vi "Create End-of-shift Report.vi"(6 "Tesla per Amp":dbl format="%#_13g", 7 "MV/m per Probe Volt":dbl format="%#_13g", 8 "error in (no error)":errorcluster, 10 "Shift Start Time":T1, 11 "Parsed Pulse Data":T2(array[cluster])) -> (0 "error out":errorcluster, 3 "Log Entry Text":string)   [LabVIEW 2013, in "Controls Log Monitor.lvlib"]
uses:
  Controls Log Monitor.lvlib
  <vilib>/Utility/miscctls.llb/LVDateTimeRec.ctl
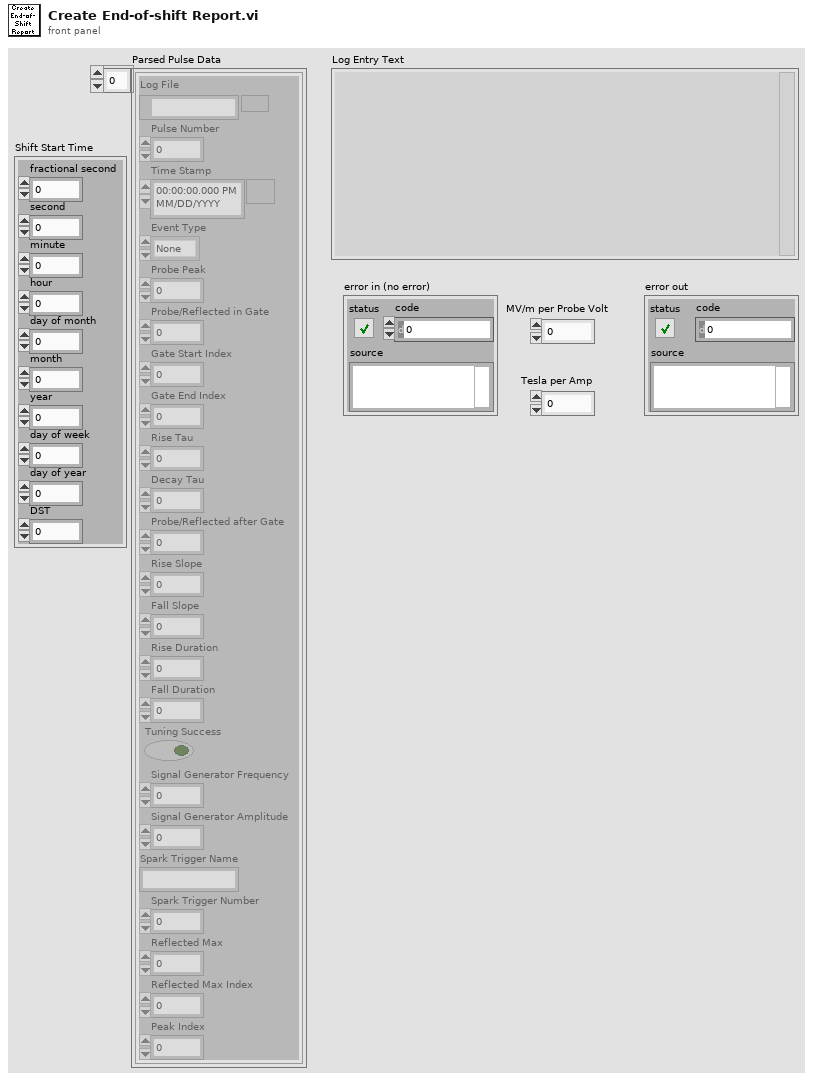
[diagram p1: front panel]
types:
  T1 = typedef "LVDateTimeRec.ctl" = cluster{"fractional second":dbl, "second":i32, "minute":i32, "hour":i32, "day of month":i32, "month":i32, "year":i32, "day of week":i32, "day of year":i32, "DST":i32}
  T2 = cluster{"Log File":path, "Pulse Number":u32, "Time Stamp":timestamp, "Event Type":enum16{"None", "Tune", "Periodic Capture", "Spark Trigger"}, "Probe Peak":dbl, "Probe/Reflected in Gate":dbl, "Gate Start Index":i32, "Gate End Index":i32, "Rise Tau":dbl, "Decay Tau":dbl, "Probe/Reflected after Gate":dbl, "Rise Slope":dbl, "Fall Slope":dbl, "Rise Duration":dbl, "Fall Duration":dbl, "Tuning Success":bool, "Signal Generator Frequency":dbl, "Signal Generator Amplitude":dbl, "Spark Trigger Name":string, "Spark Trigger Number":i32, "Reflected Max":dbl, "Reflected Max Index":i32, "Peak Index":i32}[]
  T3 = enum16{"None", "Tune", "Periodic Capture", "Spark Trigger"}
  T4 = cluster{"Name":string, "Value":dbl, "Units":string}
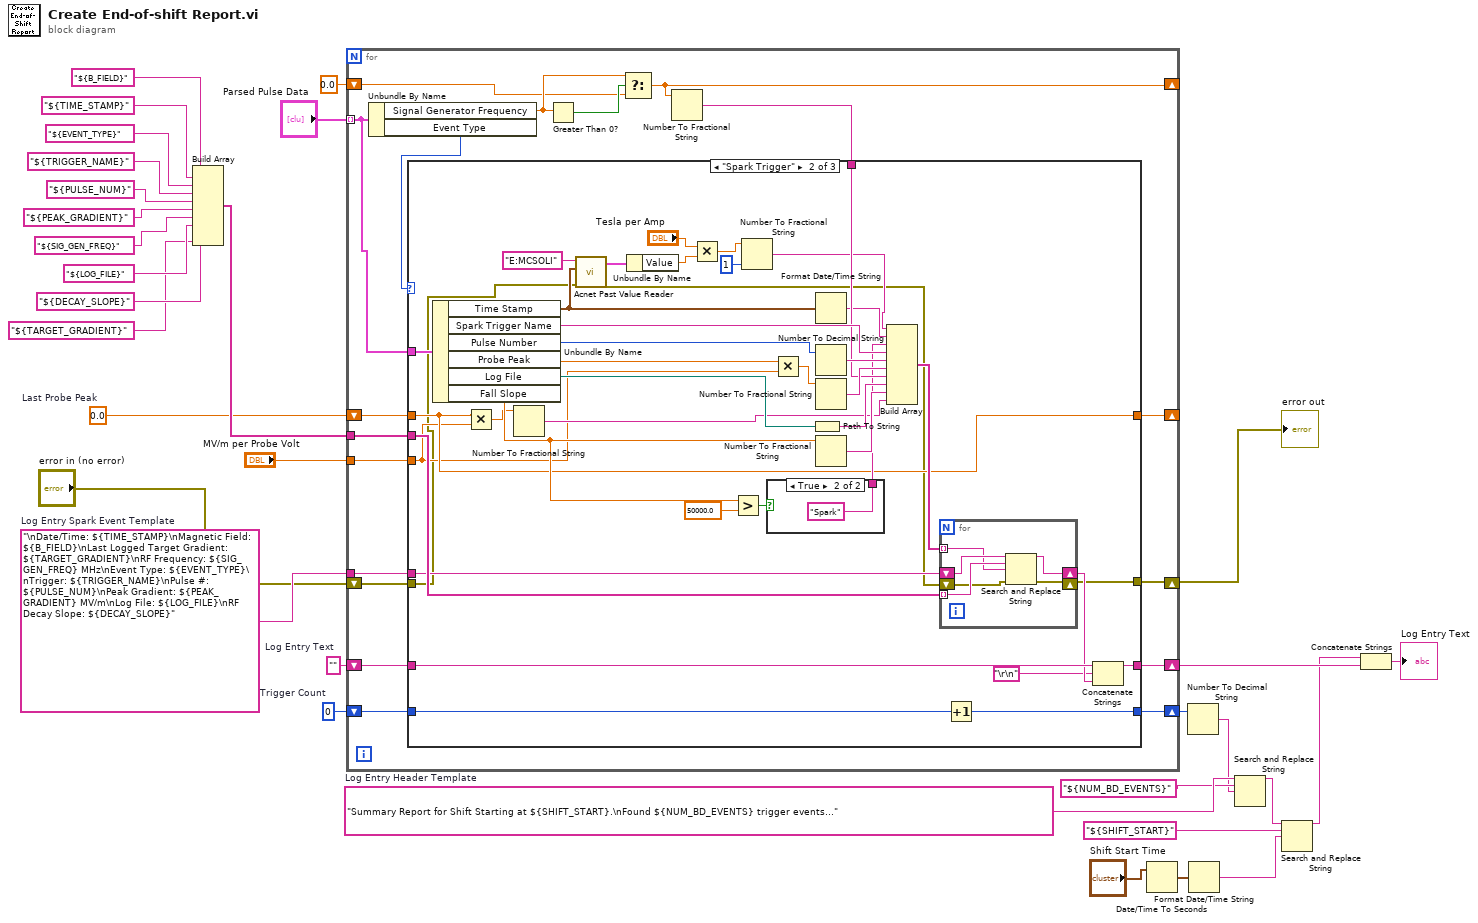
[diagram p0: block diagram]
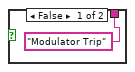
[diagram p3: hidden frame]
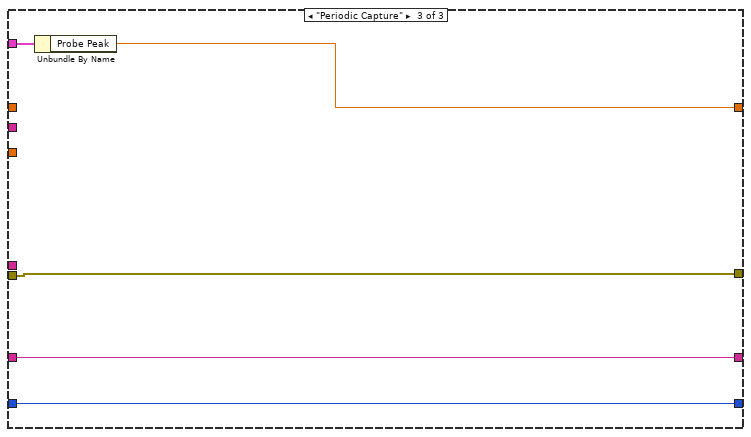
[diagram p4: hidden frame]
diagram:
  w9 = 0.0  # Last Probe Peak
  w27 = "Summary Report for Shift Starting at ${SHIFT_START}.\nFound ${NUM_BD_EVENTS} trigger events..."  # Log Entry Header Template
  w29 = ""  # Log Entry Text
  w30 = "\nDate/Time: ${TIME_STAMP}\nMagnetic Field: ${B_FIELD}\nLast Logged Target Gradient: ${TARGET_GRADIENT}\nRF Frequency: ${SIG_GEN_FREQ} MHz\nEvent Type: ${EVENT_TYPE}\nTrigger: ${TRIGGER_NAME}\nPulse #: ${PULSE_NUM}\nPeak Gradient: ${PEAK_GRADIENT} MV/m\nLog File: ${LOG_FILE}\nRF Decay Slope: ${DECAY_SLOPE}"  # Log Entry Spark Event Template
  w31 = 0  # Trigger Count
  n1 = Build Array("${B_FIELD}" ("element"), "${TIME_STAMP}" ("search string"), "${EVENT_TYPE}" ("search string"), "${TRIGGER_NAME}" ("search string"), "${PULSE_NUM}" ("search string"), "${PEAK_GRADIENT}" ("search string"), "${SIG_GEN_FREQ}" ("search string"), "${LOG_FILE}" ("search string"), "${DECAY_SLOPE}" ("search string"), "${TARGET_GRADIENT}" ("element")) -> (w16:string[])
  n2 = for {
    tunnel: "Parsed Pulse Data" -> [w48] mode=indexing
    shift-right: [w49] -> w28
    shift-left: w31 -> [w50]
    tunnel: w30 -> [w47]
    shift-right: [w41] -> w15
    shift-left: w29 -> [w46]
    shift-right: [w40] -> _
    shift-left: 0.0 ("Signal Generator Frequency") -> [w43]
    tunnel: w16 -> [w42]
    tunnel: "MV/m per Probe Volt" -> [w36]
    shift-right: [w34] -> _
    shift-left: w9 -> [w33]
    shift-right: [w37] -> w10
    shift-left: "error in (no error)" -> [w38]
    n3 = Unbundle By Name(w48) -> ("Signal Generator Frequency"=w44:dbl, "Event Type"=w35:T3)
    n4 = Greater Than 0?(x=w44) -> (x > 0?=w45:bool)
    n5 = Select(t=w44, s=w45, f=w43) -> (s? t:f=w40:dbl)
    n6 = Number To Fractional String(number=w40) -> (F-format string=w39:string)  [unwired: 3 in]
    n7 = case shown="\"Spark Trigger\"" w35 {
      tunnel: w50 -> [w54 w94 w103]
      tunnel: [w54 w93 w103] -> w49
      tunnel: w48 -> [_ w92 w107]
      tunnel: w47 -> [_ w84 _]
      tunnel: w46 -> [w53 w83 w104]
      tunnel: w42 -> [_ w85 _]
      tunnel: [w53 w82 w104] -> w41
      tunnel: w39 -> [_ w78 _]
      tunnel: w38 -> [w52 w62 w105]
      tunnel: [w52 w71 w105] -> w37
      tunnel: w36 -> [_ w65 _]
      tunnel: [w51 w66 w106] -> w34
      tunnel: w33 -> [w51 w66 _]
      frame "None", Default {
      }
      frame "Spark Trigger" {
        n8 = Unbundle By Name(w92) -> ("Time Stamp"=w64:timestamp, "Spark Trigger Name"=w89:string, "Pulse Number"=w90:u32, "Probe Peak"=w70:dbl, "Log File"=w91:path, "Fall Slope"=w75:dbl)
        n9 = Multiply(x=w66, y=w65) -> (x*y=w67:dbl)
        n10 = Number To Fractional String(number=w67) -> (F-format string=w68:string)  [unwired: 3 in]
        n11 = call "Acnet Past Value Reader.vi"("error in (no error)"=w62, "Time Stamp"=w64, "Device"="E:MCSOLI") -> ("error out"=w55:errorcluster, "Reading"=w61:T4)  [unwired: 7 in]
        n12 = Unbundle By Name(w61) -> ("Value"=w60:dbl)
        n13 = Multiply(x="Tesla per Amp", y=w60) -> (x*y=w58:dbl)
        n14 = Greater?(x=w75, y=50000.0) -> (0:w73:bool)
        n15 = Number To Fractional String(number=w58, precision (6)=i16 1) -> (F-format string=w57:string)  [unwired: 2 in]
        n16 = case shown="True" w73 {
          tunnel: ["Modulator Trip" "Spark"] -> w72
          frame False {
          }
          frame True {
          }
        }
        n17 = Multiply(x=w70, y=w65) -> (x*y=w69:dbl)
        n18 = Path To String(path=w91) -> (string=w79:string)
        n19 = Format Date/Time String(seconds (now)=w64) -> (date/time string=w77:string)  [unwired: 2 in]
        n20 = Number To Decimal String(number=w90) -> (decimal integer string=w87:string)  [unwired: 1 in]
        n21 = Number To Fractional String(number=w69) -> (F-format string=w88:string)  [unwired: 3 in]
        n22 = Number To Fractional String(number=w75) -> (F-format string=w76:string)  [unwired: 3 in]
        n23 = Build Array(w57, w77, w72, w89, w87, w88, w78, w79, w76, w68) -> (w86:string[])
        n24 = for {
          tunnel: w86 -> [w100] mode=indexing
          tunnel: w85 -> [w101] mode=indexing
          shift-right: [w99] -> w81
          shift-left: w84 -> [w102]
          shift-right: [w97] -> w71
          shift-left: w55 -> [w98]
          n25 = Search and Replace String(input string=w102, search string=w101, replace string=w100, error in=w98) -> (result string=w99:string, error out=w97:errorcluster)  [unwired: 4 in, 2 out]
        }
        n26 = Increment(x=w94) -> (x+1=w93:i32)
        n27 = Concatenate Strings(w83, "\r\n", w81) -> (w82:string)
      }
      frame "Periodic Capture" {
        n28 = Unbundle By Name(w107) -> ("Probe Peak"=w106:dbl)
      }
    }
  }
  "error out" <- w10
  n29 = Date/Time To Seconds(2:"Shift Start Time") -> (0:w3:timestamp)  [unwired: 1 in]
  n30 = Number To Decimal String(number=w28) -> (decimal integer string=w25:string)  [unwired: 1 in]
  n31 = Format Date/Time String(seconds (now)=w3) -> (date/time string=w2:string)  [unwired: 2 in]
  n32 = Search and Replace String(input string=w27, search string="${NUM_BD_EVENTS}", replace string=w25) -> (result string=w6:string)  [unwired: 5 in, 3 out]
  n33 = Search and Replace String(input string=w6, search string="${SHIFT_START}", replace string=w2) -> (result string=w1:string)  [unwired: 5 in, 3 out]
  n34 = Concatenate Strings(w1, w15) -> (→"Log Entry Text":string)
